vi "6592R_p2p_IQ_gen_1_6GHz_max.vi"() -> ()   [LabVIEW 2021]
uses:
  <vilib>/Platform/TimedLoop/XDataNode/timing_clust.ctl
  <vilib>/Platform/TimedLoop/XDataNode/nitl_modes.ctl
  <vilib>/Platform/TimedLoop/XDataNode/wakeup.ctl
  <vilib>/rvi/Emulation/niFpgaSctlEmulationGetInTimedLoop.vi
  <vilib>/rvi/Emulation/niFpgaEmulationReportErrorSimple.vi
  <vilib>/rvi/Emulation/niFpgaGetClockAttributes.vi
  <vilib>/rvi/Emulation/niFpgaCriticalErrorInLSC.vi
  <vilib>/rvi/interface/RandomDataEmulation/nirviRandomDataMultiElementFPGAFIFO.vi
  <instcachedir>/0/nirviRandomDataMultiElementFPGAFIFO_3E9965BA1FAD4E7B8DABA31768A09B1F.lvgen/nirviRandomDataMultiElementFPGAFIFO_3E9965BA1FAD4E7B8DABA31768A09B1F_000.vi
  <vilib>/rvi/interface/RandomDataEmulation/niFpgaRandomDataHandleErrors.vi
  <instrlib>/_niInstr/Basic Elements/v1/FPGA/Private/Count Up U32.vi
  <vilib>/Platform/TimedLoop/XDataNode/XDataNode.xnode
  <vilib>/rvi/DataTransferAndStorage/Container/XNode/niFpgaContainer.xnode
  <vilib>/rvi/FIFO/Fifo_Resource/nirvififoEmulationP2P.vi
  <vilib>/rvi/interface/RandomDataEmulation/nirviRandomDataFpgaMultiElementTemplate.vi
  <vilib>/Platform/TimedLoop/XDataNode/XDNodeRunTimeDep.lvlib
  <instrlib>/_niInstr/Basic Elements/v1/FPGA/niInstr Basic Elements v1 FPGA.lvlib
panel:
  out "lost sampels":u32
  in  "P2P empty room for runing":u32=2000
  out "pulse TX status":T1
  in  "reset system clock":bool
  # "Data Path Configuration"
  # "AI Trigger Configuration"
  # "AI Stream Configuration"
  # "AO Stream Configuration"
  # "Module Status"
  # "AO Buffer Configuration"
  # "Device Utilization\n---------------------------\nTotal Slices: 62.6% (18977 out of 30300)\nSlice Registers: 23.8% (115206 out of 484800)\nSlice LUTs: 38.2% (92532 out of 242400)\nBlock RAMs: 56.8% (341 out of 600)\nDSP48s: 0.3% (6 out of 1920)\n\nNote: Utilization numbers are for the KU040. Exact values will vary for the KU060 and KU035."
  # "User-defined Controls"
  # "AO Trigger Configuration"
  # "Utilization numbers are for the KU060."
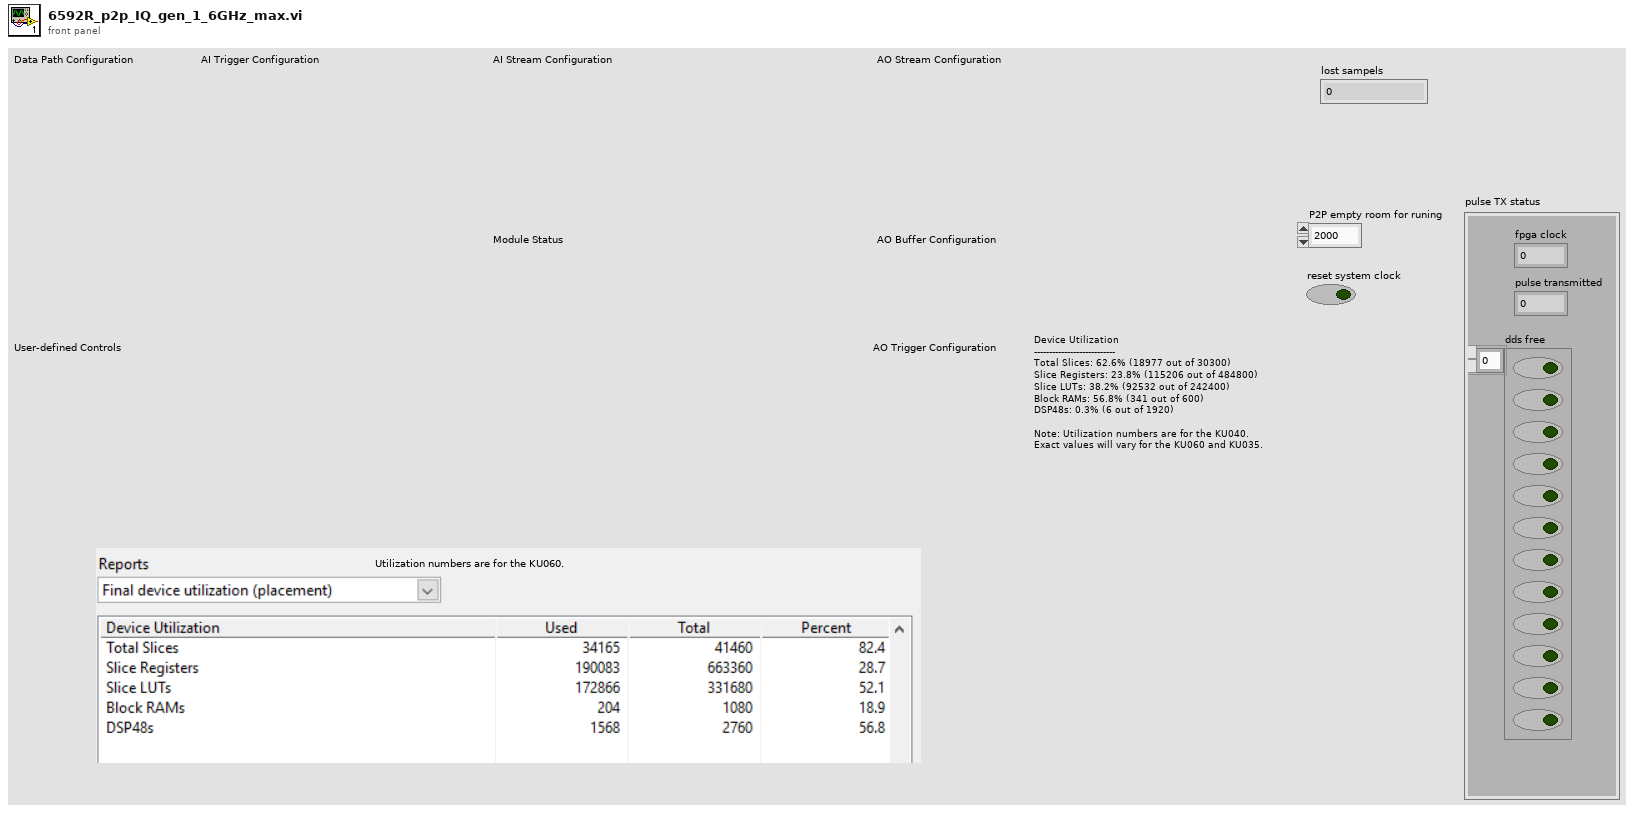
[diagram p1: front panel]
types:
  T1 = cluster{"fpga clock":u64, "pulse transmitted":u32, "dds free":bool[]}
  T2 = typedef "XDNodeRunTimeDep.lvlib/timing_clust.ctl" = cluster{"Expected End [f-1]":u64, "Actual End [f-1]":u64, "Finished Late? [f-1]":bool, "Expected End [i-1]":u64, "Actual End [i-1]":u64, "Finished Late? [i-1]":bool, "Expected Start [i]":u64, "Actual Start [i]":u64, "Expected Start [f]":u64, "Actual Start [f]":u64, "Source Name":string, "Structure Name":string, "Period":i64, "Deadline":i64, "Offset":i64, "Start":i64, "Priority":i32, "Timeout":i32, "Mode":T3, "Wakeup Reason":T4, "Error":errorcluster, "Source Type":string, "Secondary Source Type":string, "Global End Time":u64, "Global Start Time":u64, "Frame Duration":u64, "Iteration Duration":u64, "Assigned CPU":i32, "I/O Scan Engine Mode":u32}
  T3 = typedef "XDNodeRunTimeDep.lvlib/nitl_modes.ctl" = enum32{"No Change", "Process missed periods, maintain original phase", "Discard missed periods, maintain original phase", "Process missed periods, ignore original phase", "Discard missed periods, ignore original phase"}
  T4 = typedef "XDNodeRunTimeDep.lvlib/wakeup.ctl" = enum32{"Normal", "Aborted", "Asynchronous wakeup", "Timing source error", "Timed loop error", "Timeout"}
  T5 = typedef "niInstr DSP v1 Shared.lvlib/IQ Data.ctl" = cluster{"I":fxp<+/-,18,1>, "Q":fxp<+/-,18,1>, "overflow":bool}
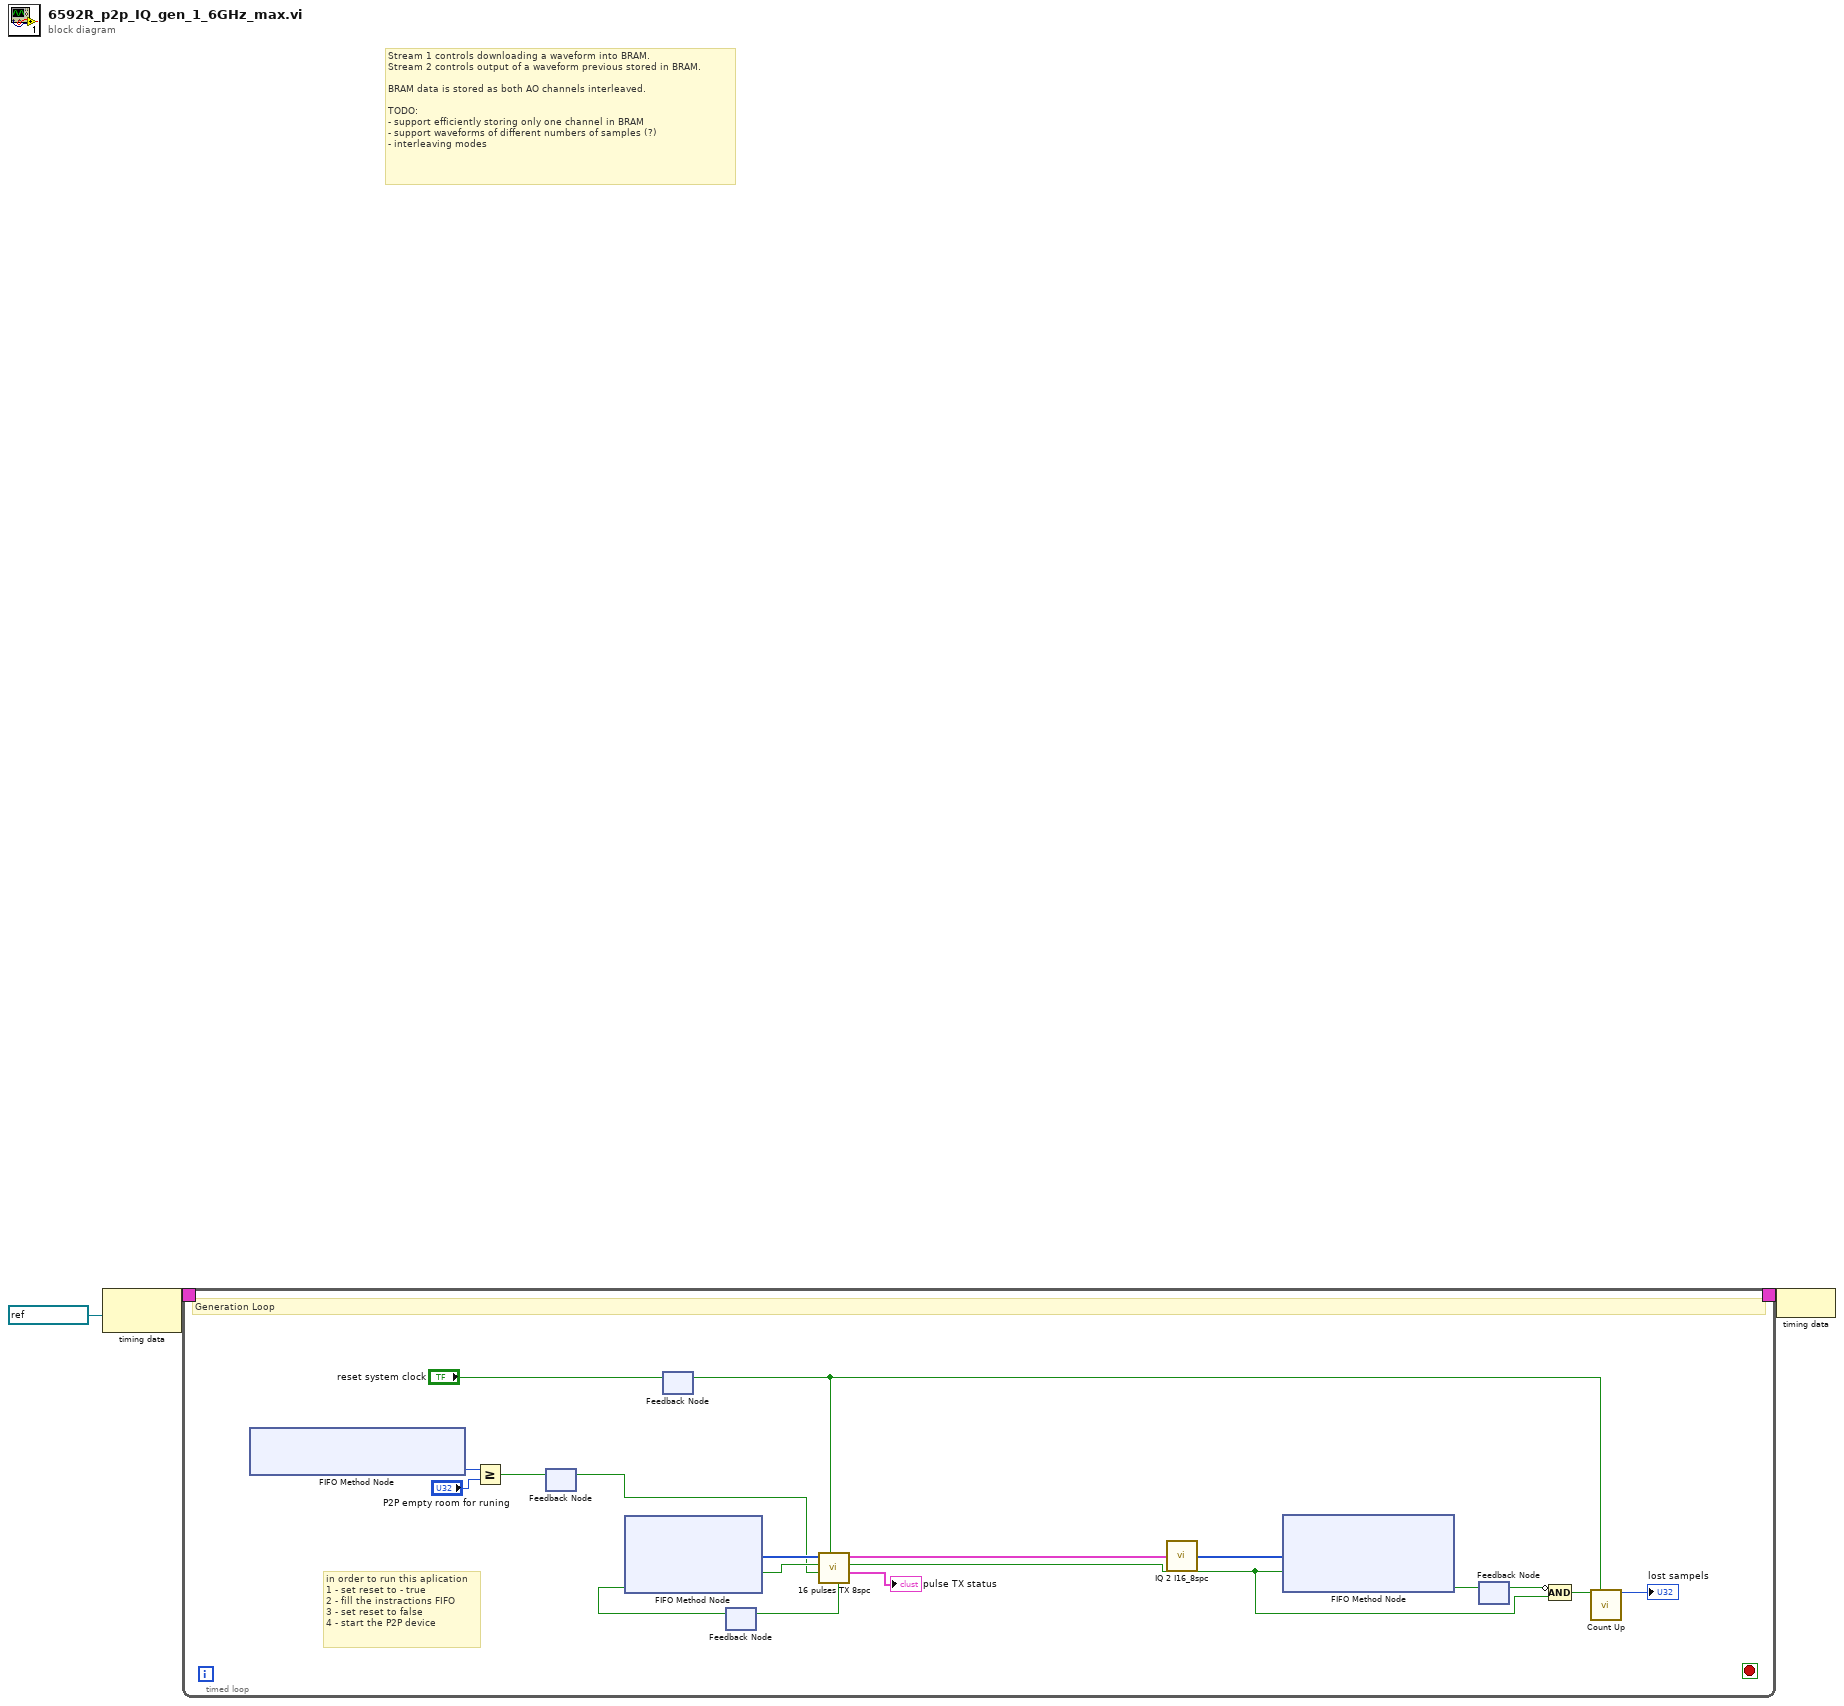
[diagram p0: block diagram]
diagram:
  # "Stream 1 controls downloading a waveform into BRAM.\nStream 2 controls output of a waveform previous stored in BRAM.\n\nBRAM data is stored as both AO channels interleaved.\n\nTODO:\n- support efficiently storing only one channel in BRAM\n- support waveforms of different numbers of samples (?)\n- interleaving modes"
  n1 = node-c288(refnum<k21> "200.1MHz" ("Source Name")) -> (w3:T2)
  n2 = timed-loop {
    timing: w3 -> [_]
    timing-out: [_] -> w2
    stop <- _ stop-if-true
    # "in order to run this aplication\n1 - set reset to - true\n2 - fill the instractions FIFO\n3 - set reset to false\n4 - start the P2P device"
    # "Generation Loop"
    n3 = xnode ("FIFO Method Node")() -> ("Number of Elements to Write"=w6:u32)  [unwired: 1 in, 1 out]
    n4 = Greater Or Equal?(x=w6, y="P2P empty room for runing") -> (x >= y?=w15:bool)
    n5 = feedback #1() -> (w16:bool)  [unwired: 1 in]
    n6 = feedback-in #1(w15) -> ()
    n7 = feedback-in #2("reset system clock") -> ()
    n8 = feedback #2() -> (w10:bool)  [unwired: 1 in]
    n9 = feedback #3() -> (w20:bool)  [unwired: 1 in]
    n10 = xnode ("FIFO Method Node")("Ready for Output"=w20) -> ("Element"=w19:u64[], "Output Valid"=w18:bool)  [unwired: 1 in, 1 out]
    n11 = call "16 pulses TX 8spc.vi"("reset system clock"=w10, "IQ_run"=w16, "PDW input Valid"=w18, "array PDW"=w19) -> ("pulse TX status"=→"pulse TX status":T1, "output valid"=w4:bool, "IQ out"=w5:T5[], "ready for input"=w21:bool)  [unwired: 4 in]
    n12 = feedback-in #3(w21) -> ()
    n13 = call "IQ 2 I16_8spc.vi"("IQ in"=w5) -> ("interleaved IQ array"=w8:i16[])
    n14 = xnode ("FIFO Method Node")("Element"=w8, "Input Valid"=w4) -> ("Ready for Input"=w7:bool)  [unwired: 1 in, 1 out]
    n15 = feedback-in #4(w7) -> ()
    n16 = feedback #4() -> (w13:bool)  [unwired: 1 in]
    n17 = Compound Arithmetic op=AND(invert w13, w4) -> (w12:bool)
    n18 = call-poly <instrlib>:"Count Up.vi"("increment"=w12, "reset"=w10) -> ("count out"=→"lost sampels":u32)  [unwired: 13 in]
  }
  n19 = node-c288(w2) -> ()
